vi "Sekunden seit Tagesbeginn.vi"(7 "in":dbl[](array[numeric])) -> (8 "out":dbl[](array[numeric]))   [LabVIEW 2017, in "util.lvlib"]
uses:
  util.lvlib
  <vilib>/Utility/miscctls.llb/LVDateTimeRec.ctl
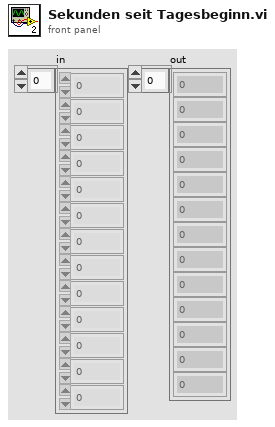
[diagram p1: front panel]
types:
  T1 = typedef "LVDateTimeRec.ctl" = cluster{"fractional second":dbl, "second":i32, "minute":i32, "hour":i32, "day of month":i32, "month":i32, "year":i32, "day of week":i32, "day of year":i32, "DST":i32}
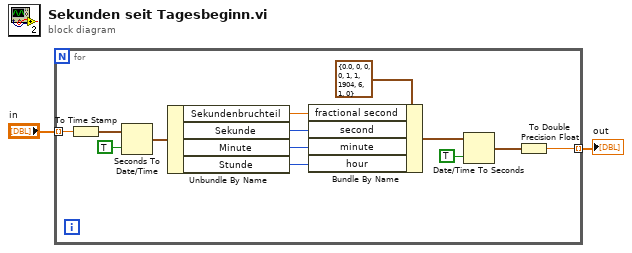
[diagram p0: block diagram]
diagram:
  n1 = for {
    tunnel: "in" -> [w14] mode=indexing
    tunnel: [w3] -> w1 mode=indexing
    n2 = To Time Stamp(1:w14) -> (0:w4:timestamp)
    n3 = Seconds To Date/Time(time stamp (now)=w4, to UTC (F)=TRUE ("in Weltzeit (F)")) -> (date time rec=w6:T1)
    n4 = Unbundle By Name(w6) -> ("Sekundenbruchteil"=w8:dbl, "Sekunde"=w9:i32, "Minute"=w10:i32, "Stunde"=w11:i32)
    n5 = Bundle By Name(cluster=T1 {"fractional second"=0.0, "second"=0, "minute"=0, "hour"=0, "day of month"=1, "month"=1, "year"=1904, "day of week"=6, "day of year"=1, "DST"=0} ("Datum/Zeit"), "fractional second"=w8, "second"=w9, "minute"=w10, "hour"=w11) -> (w12:T1)
    n6 = Date/Time To Seconds(1:TRUE ("Weltzeit (F)"), 2:w12) -> (0:w5:timestamp)
    n7 = To Double Precision Float(number=w5) -> (double precision float=w3:dbl)
  }
  "out" <- w1
